vi "TrajectoryGetClosedLoop.vi"() -> (3 "AUTO_CLOSED_LOOP":bool)   [LabVIEW 2023]
uses:
  TrajectoryGlobals.vi
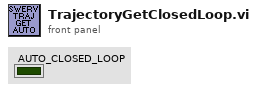
[diagram p1: front panel]
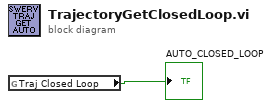
[diagram p0: block diagram]
diagram:
  n1 = global read "TrajectoryGlobals.vi" "Traj Closed Loop"() -> (→"AUTO_CLOSED_LOOP":bool)
